vi "项目输入.vi"() -> (1 "输入有效":bool, 2 "项目名称":string)   [LabVIEW 2013]
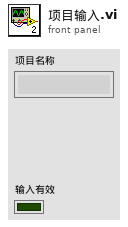
[diagram p1: front panel]
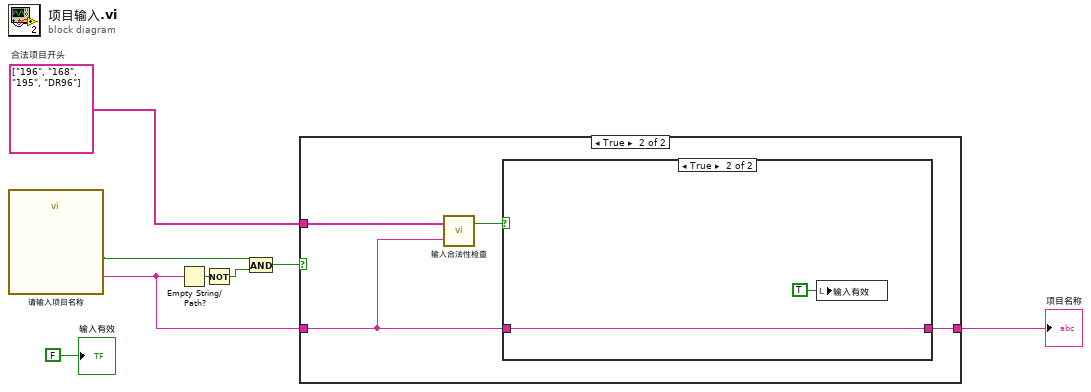
[diagram p0: block diagram]
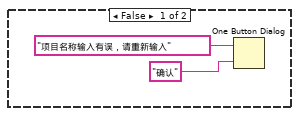
[diagram p3: hidden frame]
diagram:
  w3 = string[] ["196", "168", "195", "DR96"]  # 合法项目开头
  n1 = call "请输入项目名称"() -> ("项目名称"=w4:string, "确认"=w6:bool)  [unwired: 17 in, 1 out]
  n2 = Empty String/Path?(string/path=w4) -> (empty?=w8:bool)
  n3 = Not(x=w8) -> (.not. x?=w7:bool)
  n4 = And(x=w6, y=w7) -> (x .and. y?=w5:bool)
  n5 = case shown="True" w5 {
    tunnel: w4 -> [_ w9]
    tunnel: w3 -> [_ w11]
    tunnel: [_ w10] -> w2
    frame False {
    }
    frame True {
      n6 = call "输入合法性检查.vi"("被检查名称"=w9, "合法名称集合"=w11) -> ("输入有效"=w12:bool)  [unwired: 1 out]
      n7 = case shown="True" w12 {
        tunnel: [_ w16] -> w10
        tunnel: w9 -> [_ w16]
        frame False {
          n8 = One Button Dialog(message="项目名称输入有误，请重新输入", button name ("OK")="确认") -> ()  [unwired: 1 out]
        }
        frame True {
          n9 = local write "输入有效"(TRUE ("输入有效")) -> ()
        }
      }
    }
  }
  "项目名称" <- w2
  "输入有效" <- FALSE
